vi "SMO.UI.Example.Get Dependencies.vi"(8 "error in (no error)":errorcluster, 11 "SMO UI.Template in":refnum<class "SMO.UI.Example.lvclass">) -> (0 "error out":errorcluster, 2 "Dependencies":T1, 3 "SMO UI.Template out":refnum<class "SMO.UI.Example.lvclass">)   [LabVIEW 2013, in "SMO.UI.Example.lvclass"]
uses:
  SMO.UI.Example.lvclass
  Typedefs/Dependencies--Cluster.ctl
  SMO.Example/SMO.Example.lvclass
  SMO/SMO.lvclass
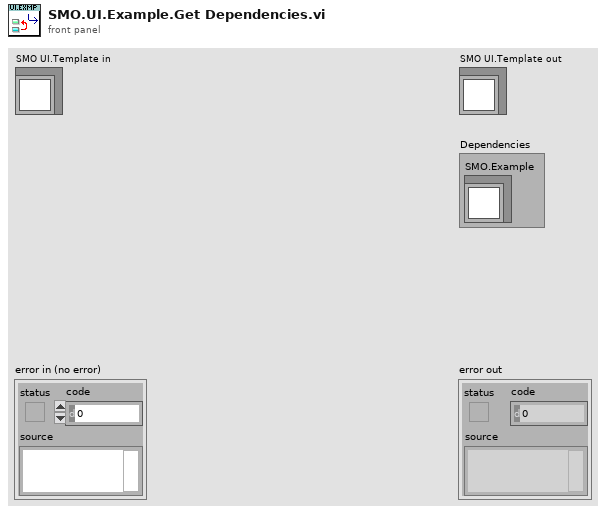
[diagram p1: front panel]
types:
  T1 = typedef "SMO.UI.Example.lvclass/Dependencies--Cluster.ctl" = cluster{"SMO.Example":refnum<class "SMO.Example.lvclass">}
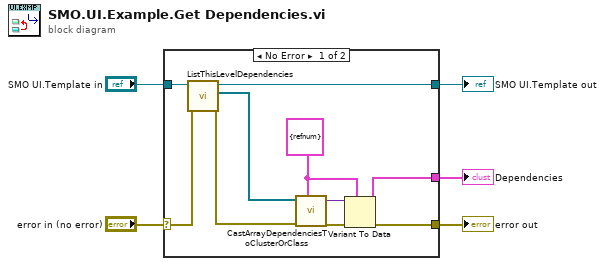
[diagram p0: block diagram]
diagram:
  n1 = case shown="No Error" "error in (no error)" {
    selector: "error in (no error)" -> [w7 w16]
    tunnel: [w6 w16] -> w4
    tunnel: [w10 w17] -> w2
    tunnel: "SMO UI.Template in" -> [w11 w17]
    tunnel: [w8 _] -> w1
    frame No Error {
      w9 = T1 {"SMO.Example"=refnum} ("Dependencies")
      n2 = call "ListThisLevelDependencies.vi"("error in (no error)"=w7, "SMO in"=w11) -> ("error out"=w12:errorcluster, "[My Dependencies]"=w15:refnum<class "SMO.lvclass">[], "SMO out"=w10:refnum<class "SMO.UI.Example.lvclass">)  [unwired: 7 in]
      n3 = call "CastArrayDependenciesToClusterOrClass.vi"("Dependency Type (Class|Cluster)"=w9, "error in (no error)"=w12, "[Dependencies]"=w15) -> ("error out"=w14:errorcluster, "Dependencies output"=w13:variant)  [unwired: 7 in]
      n4 = Variant To Data(error in=w14, type=w9, Variant=w13) -> (data=w8:T1, error out=w6:errorcluster)
    }
    frame Error {
    }
  }
  "error out" <- w4
  "SMO UI.Template out" <- w2
  "Dependencies" <- w1
